vi "Enable Control.vi"(7 "Select Channel":i32=1 min=1 max=4 step=1, 8 "error in (no error)":errorcluster, 10 "Enable Control":bool, 11 "Lakeshore 325 in":refnum<class "Lakeshore 325.lvclass">) -> (0 "error out":errorcluster, 3 "Lakeshore 325 out":refnum<class "Lakeshore 325.lvclass">)   [LabVIEW 2022 SP3, in "Lakeshore 325.lvclass"]
uses:
  Lakeshore 325.lvclass
  Lakeshore 325.lvclass/Lakeshore 325.ctl
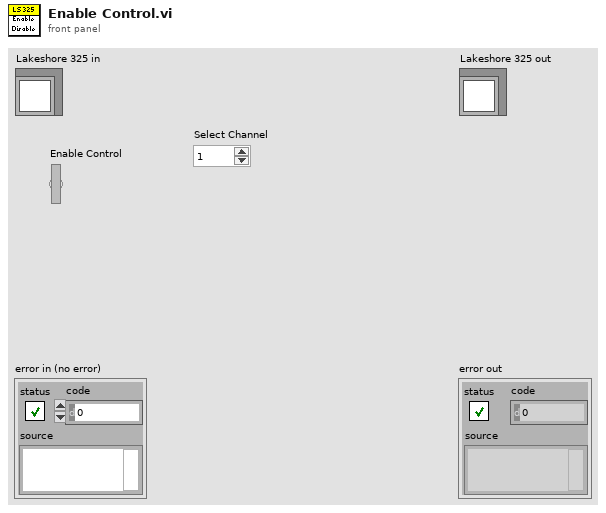
[diagram p1: front panel]
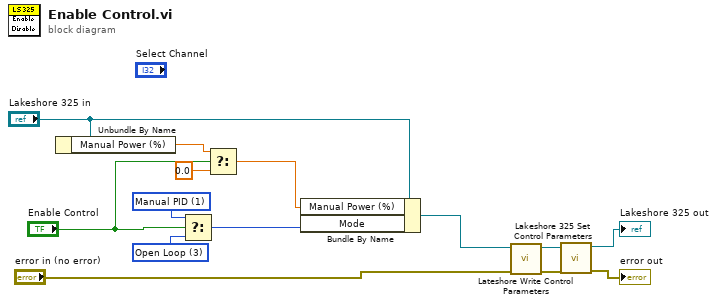
[diagram p0: block diagram]
diagram:
  w13 = u16 3 items=["Manual PID"=1, "Zone"=2, "Open Loop"=3, "AutoTune PID"=4, "AutoTune PI"=5, "AutoTune P"=6] ("Mode (1:Manual PID)")
  w14 = u16 1 items=["Manual PID"=1, "Zone"=2, "Open Loop"=3, "AutoTune PID"=4, "AutoTune PI"=5, "AutoTune P"=6] ("Mode (1:Manual PID)")
  n1 = Unbundle By Name("Lakeshore 325 in") -> ("Manual Power (%)"=w9:dbl)
  n2 = Select(t=w14, s="Enable Control", f=w13) -> (s? t:f=w12:u16)
  n3 = Select(t=w9, s="Enable Control", f=0.0) -> (s? t:f=w7:dbl)
  n4 = Bundle By Name(cluster="Lakeshore 325 in", "Manual Power (%)"=w7, "Mode"=w12) -> (w4:refnum<class "Lakeshore 325.lvclass">)
  n5 = call "Lateshore Write Control Parameters.vi"("error in (no error)"="error in (no error)", "Lakeshore 325 in"=w4) -> ("error out"=w1:errorcluster, "Lakeshore 325 out"=w3:refnum<class "Lakeshore 325.lvclass">)  [unwired: 8 in]
  n6 = call "Lakeshore 325 Set Control Parameters.vi"("error in (no error)"=w1, "Lakeshore 325 in"=w3) -> ("error out"=→"error out":errorcluster, "Lakeshore 325 out"=→"Lakeshore 325 out":refnum<class "Lakeshore 325.lvclass">)  [unwired: 8 in]
